vi "TDMS_DataHandler_Create.vi"(0 "reference in":refnum<class "TDMS_DataHandler.lvclass">, 1 "TDMS file path":path, 2 "Group name":string="Force Curve", 5 "error in (no error)":errorcluster, 7 "object name":string) -> (14 "reference out":refnum<class "TDMS_DataHandler.lvclass">, 19 "error out":errorcluster)   [LabVIEW 2019, in "TDMS_DataHandler.lvclass"]
doc: "Constructor."
uses:
  TDMS_DataHandler.lvclass
  C:/Program Files/National Instruments/LabVIEW 2019/vi.lib/addons/_AddQ/G#Object/G#Object.lvclass
  <vilib>/addons/_AddQ/G#Object/G#Object.lvclass
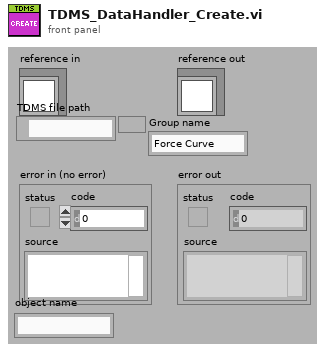
[diagram p1: front panel]
types:
  T1 = typedef "TDMS_DataHandler.lvclass/ObjectAttributesRef.ctl" = refnum<data-value>
  T2 = typedef "TDMS_DataHandler.lvclass/ObjectAttributes.ctl" = cluster{"Directory":path, "FilePath":path, "FileRef":refnum<k34>, "ExperimentName":string, "GroupName":string, "ChannelNames":string[], "Datum":waveform(dbl)[], "Group_Metadata":cluster{"property names":string[], "property values":variant[]}, "Channel_Metadata":cluster{"property names":string[], "property values":variant[]}}
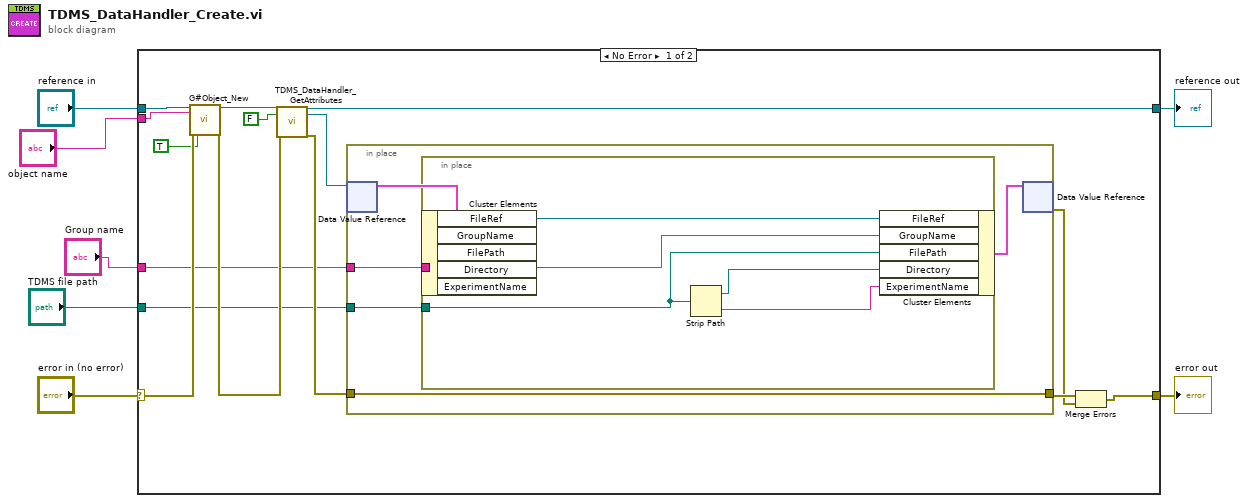
[diagram p0: block diagram]
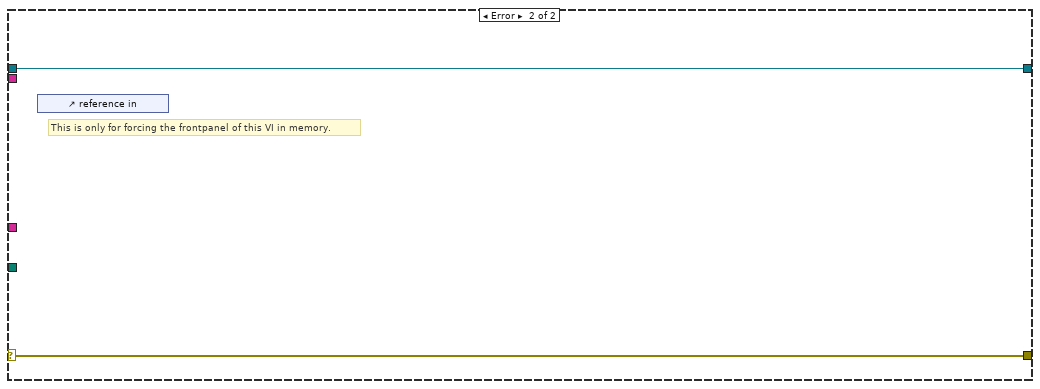
[diagram p2: hidden frame]
diagram:
  n1 = case shown="No Error" "error in (no error)" {
    selector: "error in (no error)" -> [w21 w34]
    tunnel: [w20 w34] -> w6
    tunnel: [w15 w33] -> w4
    tunnel: "reference in" -> [w22 w33]
    tunnel: "TDMS file path" -> [w10 _]
    tunnel: "Group name" -> [w9 _]
    tunnel: "object name" -> [w8 _]
    frame No Error {
      n2 = call <vilib>:"G#Object_New.vi"("reference in"=w22, "object name"=w8, "error in (no error)"=w21, "user counter (T)?"=TRUE ("User Counter")) -> ("reference out"=w16:refnum<class "TDMS_DataHandler.lvclass">, "error out"=w14:errorcluster)  [unwired: 13 in, 1 out]
      n3 = call "TDMS_DataHandler_GetAttributes.vi"("reference in"=w16, "return data? (T)"=FALSE ("return data"), "error in (no error)"=w14) -> ("reference out"=w15:refnum<class "TDMS_DataHandler.lvclass">, "attributes ref"=w13:T1, "error out"=w11:errorcluster)  [unwired: 13 in, 1 out]
      n4 = in-place {
        in-place-border: w11 -> [w25]
        in-place-border: [w25] -> w18
        in-place-border: w10 -> [w24]
        in-place-border: w9 -> [w23]
        n5 = in-place-dvr #1(w13) -> (w26:T2)  [unwired: 1 out]
        n6 = in-place {
          in-place-border: w24 -> [w30]
          in-place-border: w23 -> [w31]
          n7 = in-place-cluster #2(w26) -> ("FileRef"=w32:refnum<k34>)  [unwired: 4 out]
          n8 = Strip Path(path=w30) -> (stripped path=w29:path, name=w28:string)
          n9 = in-place-cluster #2("FileRef"=w32, "GroupName"=w31, "FilePath"=w30, "Directory"=w29, "ExperimentName"=w28) -> (w27:T2)
        }
        n10 = in-place-dvr #1(w27) -> (w17:errorcluster)  [unwired: 1 out]
      }
      n11 = Merge Errors(w18, w17) -> (w20:errorcluster)
    }
    frame Error {
      # "This is only for forcing the frontpanel of this VI in memory."
      n12 = control-ref of="reference in"() -> ()  [unwired: 1 out]
    }
  }
  "error out" <- w6
  "reference out" <- w4
